vi "TREE_color selector.vi"(8 "error in":errorcluster, 10 "Selector color":u32(colorbox)=15925199, 11 "Tree In":refnum<vi>) -> (0 "error out":errorcluster, 3 "Tree Out":refnum<vi>)   [LabVIEW 2011]
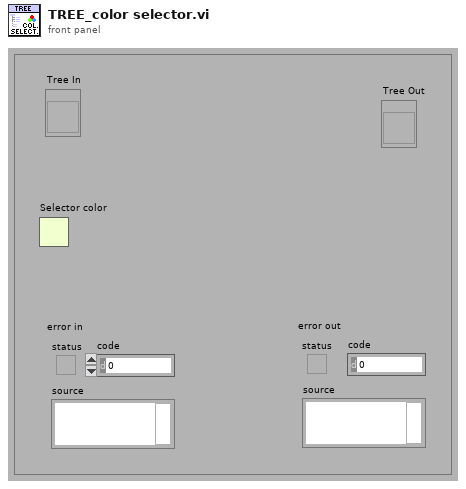
[diagram p1: front panel]
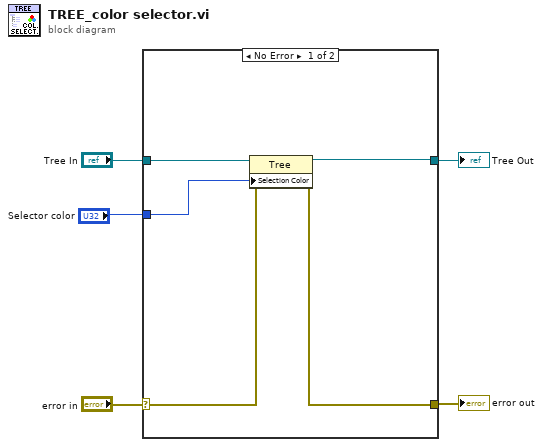
[diagram p0: block diagram]
diagram:
  n1 = case shown="No Error" "error in" {
    selector: "error in" -> [w10 w12]
    tunnel: "Tree In" -> [w9 w11]
    tunnel: [w7 w11] -> w4
    tunnel: [w8 w12] -> w3
    tunnel: "Selector color" -> [w6 _]
    frame No Error {
      n2 = property class="Tree"(reference=w9, error in=w10, "Selection Color"=w6) -> (reference out=w7:refnum<vi>, error out=w8:errorcluster)
    }
    frame Error {
      (unwired) string[] [] ("directory names")
      (unwired) path ""
      (unwired) "" ("name")
    }
  }
  "Tree Out" <- w4
  "error out" <- w3
